vi "IMS Stepper -- V4.vi"() -> ()   [LabVIEW 2018]
doc: "Use this template to build a producer/consumer design pattern with events to produce queue items. Use this design pattern instead of the User Interface Event Handler pattern for user interfaces when you want to execute code asynchronously in response to an event without slowing the user interface responsiveness."
uses:
  publisher action.ctl
  motor internal action.ctl
  slider action.ctl
  slider setter action.ctl
  stepper motor action.ctl
  slider setter interal state.ctl
  stepper motor state.ctl
  internal stepper driver state -- IMS.ctl
  stepper monitor message.ctl
panel:
  in  "Tab Control":enum32{"main", "init&stuff", "ignore"}(tab)
  in  "speed":i32=4003
  in  "stepper state":T1=enum."stopped"
  in  "set angle":dbl(slide)=-10.106382978723403 scale=-56.0..55.0 scale format="%^#6_6g"
  in  "XY Graph":cluster{dbl[], dbl[]}[](graph)=[{[-0.30000000000000004, -0.23550000000000004, -0.17100000000000004, -0.10650000000000004, -0.04200000000000004, 0.022499999999999964, 0.08699999999999997, 0.15149999999999997, 0.21599999999999997, 0.28049999999999997, 0.345, 0.4095, 0.474, 0.5385, 0.603, 0.6675, 0.732, 0.7965, 0.861, 0.9255], [0.0, 0.0, 0.0, 0.0, 0.0, 0.0, 0.0, 0.0, 0.0, 0.0, 0.0, 0.0, 0.0, 0.0, 0.0, 0.0, 0.0, 0.0, 0.0, 0.0]}, {[-0.29607463230851366, -0.23241858636218324, -0.1687625404158528, -0.10510649446952239, -0.04145044852319196, 0.02220559742313849, 0.08586164336946889, 0.14951768931579928, 0.21317373526212974, 0.2768297812084602, 0.34048582715479064, 0.404141873101121, 0.46779791904745144, 0.531453964993782, 0.5951100109401122, 0.6587660568864426, 0.7224221028327731, 0.7860781487791035, 0.849734194725434, 0.9133902406717644], [0.048371604308503874, 0.03797170938217554, 0.02757181445584721, 0.01717191952951888, 0.006772024603190548, -0.0036278703231377857, -0.014027765249466112, -0.024427660175794452, -0.03482755510212278, -0.045227450028451105, -0.055627344954779445, -0.06602723988110777, -0.0764271348074361, -0.08682702973376444, -0.09722692466009278, -0.10762681958642109, -0.11802671451274943, -0.12842660943907777, -0.13882650436540608, -0.14922639929173442]}, {[1.0, 0.9980267284282716, 0.9921147013144779, 0.9822872507286887, 0.9685831611286311, 0.9510565162951535, 0.9297764858882513, 0.9048270524660195, 0.8763066800438636, 0.8443279255020151, 0.8090169943749475, 0.7705132427757891, 0.7289686274214116, 0.6845471059286886, 0.6374239897486896, 0.587785252292473, 0.5358267949789965, 0.48175367410171516, 0.42577929156507266, 0.36812455268467786, 0.30901699437494745, 0.24868988716485474, 0.18738131458572452, 0.12533323356430426, 0.0627905195293133, -1.6081428723391245e-16, -0.0627905195293134, -0.12533323356430437, -0.18738131458572482, -0.24868988716485485, -0.30901699437494756, -0.368124552684678, -0.4257792915650727, -0.48175367410171543, -0.5358267949789969, -0.587785252292473, -0.6374239897486897, -0.6845471059286887, -0.7289686274214117, -0.7705132427757894, -0.8090169943749473, -0.8443279255020151, -0.8763066800438636, -0.9048270524660196, -0.9297764858882515, -0.9510565162951536, -0.9685831611286311, -0.9822872507286887, -0.9921147013144779, -0.9980267284282716, -1.0, -0.9980267284282716, -0.9921147013144779, -0.9822872507286886, -0.9685831611286311, -0.9510565162951535, -0.9297764858882512, -0.9048270524660195, -0.8763066800438635, -0.844327925502015, -0.8090169943749472, -0.770513242775789, -0.7289686274214116, -0.6845471059286886, -0.6374239897486895, -0.5877852522924732, -0.5358267949789963, -0.48175367410171527, -0.42577929156507216, -0.3681245526846778, -0.30901699437494756, -0.24868988716485443, -0.18738131458572463, -0.12533323356430373, -0.06279051952931321, -1.836909530733566e-16, 0.06279051952931372, 0.12533323356430423, 0.18738131458572513, 0.24868988716485493, 0.30901699437494723, 0.36812455268467825, 0.4257792915650726, 0.4817536741017157, 0.5358267949789968, 0.5877852522924737, 0.63742398974869, 0.6845471059286886, 0.7289686274214119, 0.7705132427757894, 0.8090169943749478, 0.8443279255020153, 0.8763066800438636, 0.9048270524660197, 0.9297764858882515, 0.9510565162951538, 0.9685831611286312, 0.9822872507286887, 0.9921147013144779, 0.9980267284282716], [0.0, 0.06279051952931337, 0.12533323356430426, 0.18738131458572463, 0.2486898871648548, 0.3090169943749474, 0.368124552684678, 0.4257792915650727, 0.4817536741017153, 0.5358267949789967, 0.5877852522924731, 0.6374239897486897, 0.6845471059286887, 0.7289686274214116, 0.7705132427757893, 0.8090169943749475, 0.8443279255020151, 0.8763066800438637, 0.9048270524660196, 0.9297764858882515, 0.9510565162951535, 0.9685831611286311, 0.9822872507286887, 0.9921147013144779, 0.9980267284282716, 1.0, 0.9980267284282716, 0.9921147013144778, 0.9822872507286886, 0.9685831611286311, 0.9510565162951535, 0.9297764858882513, 0.9048270524660195, 0.8763066800438635, 0.844327925502015, 0.8090169943749475, 0.7705132427757893, 0.7289686274214114, 0.6845471059286885, 0.6374239897486895, 0.5877852522924732, 0.5358267949789967, 0.4817536741017152, 0.4257792915650725, 0.36812455268467775, 0.3090169943749471, 0.24868988716485482, 0.18738131458572457, 0.1253332335643041, 0.06279051952931314, -3.216285744678249e-16, -0.06279051952931335, -0.12533323356430429, -0.18738131458572477, -0.24868988716485502, -0.30901699437494773, -0.3681245526846783, -0.42577929156507266, -0.4817536741017154, -0.5358267949789968, -0.5877852522924734, -0.63742398974869, -0.6845471059286887, -0.7289686274214116, -0.7705132427757894, -0.8090169943749473, -0.8443279255020153, -0.8763066800438636, -0.9048270524660198, -0.9297764858882515, -0.9510565162951535, -0.9685831611286312, -0.9822872507286887, -0.9921147013144779, -0.9980267284282716, -1.0, -0.9980267284282716, -0.9921147013144779, -0.9822872507286886, -0.9685831611286311, -0.9510565162951536, -0.9297764858882512, -0.9048270524660196, -0.8763066800438634, -0.844327925502015, -0.809016994374947, -0.770513242775789, -0.7289686274214116, -0.6845471059286883, -0.6374239897486896, -0.5877852522924726, -0.5358267949789963, -0.4817536741017153, -0.4257792915650722, -0.36812455268467786, -0.3090169943749468, -0.2486898871648545, -0.18738131458572468, -0.1253332335643038, -0.06279051952931326]}, {[0.1, 0.09980267284282716, 0.0992114701314478, 0.09822872507286888, 0.09685831611286311, 0.09510565162951536, 0.09297764858882514, 0.09048270524660196, 0.08763066800438636, 0.08443279255020152, 0.08090169943749476, 0.07705132427757892, 0.07289686274214116, 0.06845471059286887, 0.06374239897486897, 0.05877852522924731, 0.05358267949789966, 0.04817536741017152, 0.042577929156507266, 0.03681245526846779, 0.030901699437494747, 0.024868988716485477, 0.018738131458572452, 0.012533323356430426, 0.006279051952931331, -1.6081428723391246e-17, -0.0062790519529313405, -0.012533323356430438, -0.018738131458572484, -0.024868988716485487, -0.030901699437494757, -0.0368124552684678, -0.04257792915650727, -0.048175367410171546, -0.05358267949789969, -0.05877852522924731, -0.06374239897486898, -0.06845471059286888, -0.07289686274214117, -0.07705132427757894, -0.08090169943749474, -0.08443279255020152, -0.08763066800438636, -0.09048270524660196, -0.09297764858882515, -0.09510565162951537, -0.09685831611286311, -0.09822872507286888, -0.0992114701314478, -0.09980267284282716, -0.1, -0.09980267284282716, -0.0992114701314478, -0.09822872507286887, -0.09685831611286311, -0.09510565162951536, -0.09297764858882512, -0.09048270524660196, -0.08763066800438635, -0.0844327925502015, -0.08090169943749473, -0.07705132427757891, -0.07289686274214116, -0.06845471059286887, -0.06374239897486896, -0.05877852522924733, -0.05358267949789963, -0.04817536741017153, -0.04257792915650722, -0.036812455268467784, -0.030901699437494757, -0.024868988716485445, -0.018738131458572463, -0.012533323356430374, -0.006279051952931321, -1.836909530733566e-17, 0.006279051952931373, 0.012533323356430424, 0.018738131458572515, 0.024868988716485494, 0.030901699437494726, 0.036812455268467825, 0.042577929156507266, 0.048175367410171574, 0.05358267949789968, 0.05877852522924737, 0.063742398974869, 0.06845471059286887, 0.07289686274214119, 0.07705132427757894, 0.08090169943749478, 0.08443279255020153, 0.08763066800438636, 0.09048270524660197, 0.09297764858882515, 0.09510565162951538, 0.09685831611286312, 0.09822872507286888, 0.0992114701314478, 0.09980267284282716], [0.0, 0.006279051952931338, 0.012533323356430426, 0.018738131458572463, 0.02486898871648548, 0.03090169943749474, 0.0368124552684678, 0.04257792915650727, 0.04817536741017153, 0.05358267949789967, 0.058778525229247314, 0.06374239897486898, 0.06845471059286888, 0.07289686274214116, 0.07705132427757894, 0.08090169943749476, 0.08443279255020152, 0.08763066800438638, 0.09048270524660196, 0.09297764858882515, 0.09510565162951536, 0.09685831611286311, 0.09822872507286888, 0.0992114701314478, 0.09980267284282716, 0.1, 0.09980267284282716, 0.09921147013144778, 0.09822872507286887, 0.09685831611286311, 0.09510565162951536, 0.09297764858882514, 0.09048270524660196, 0.08763066800438635, 0.0844327925502015, 0.08090169943749476, 0.07705132427757894, 0.07289686274214115, 0.06845471059286885, 0.06374239897486896, 0.05877852522924733, 0.05358267949789967, 0.048175367410171525, 0.04257792915650725, 0.03681245526846778, 0.030901699437494712, 0.024868988716485484, 0.01873813145857246, 0.01253332335643041, 0.0062790519529313145, -3.216285744678249e-17, -0.006279051952931335, -0.01253332335643043, -0.018738131458572477, -0.024868988716485504, -0.030901699437494774, -0.03681245526846783, -0.042577929156507266, -0.04817536741017154, -0.05358267949789968, -0.05877852522924734, -0.063742398974869, -0.06845471059286888, -0.07289686274214116, -0.07705132427757894, -0.08090169943749474, -0.08443279255020153, -0.08763066800438636, -0.09048270524660199, -0.09297764858882515, -0.09510565162951536, -0.09685831611286312, -0.09822872507286888, -0.0992114701314478, -0.09980267284282716, -0.1, -0.09980267284282716, -0.0992114701314478, -0.09822872507286887, -0.09685831611286311, -0.09510565162951537, -0.09297764858882512, -0.09048270524660196, -0.08763066800438635, -0.0844327925502015, -0.0809016994374947, -0.07705132427757891, -0.07289686274214116, -0.06845471059286883, -0.06374239897486897, -0.05877852522924726, -0.05358267949789963, -0.04817536741017153, -0.042577929156507224, -0.03681245526846779, -0.03090169943749468, -0.02486898871648545, -0.01873813145857247, -0.012533323356430379, -0.006279051952931327]}, {[0.0, 0.0, 0.0, 0.0, 0.0, 0.0, 0.0, 0.0, 0.0, 0.0, 0.0, 0.0, 0.0, 0.0, 0.0, 0.0, 0.0, 0.0, 0.0, 0.0], [1.1, 1.135, 1.1700000000000002, 1.205, 1.24, 1.2750000000000001, 1.31, 1.345, 1.3800000000000001, 1.415, 1.4500000000000002, 1.485, 1.52, 1.5550000000000002, 1.59, 1.625, 1.6600000000000001, 1.695, 1.73, 1.7650000000000001]}, {[-0.09587131702242406, -0.09674287444990064, -0.09761443187737723, -0.0984859893048538, -0.0993575467323304, -0.10022910415980697, -0.10110066158728355, -0.10197221901476014, -0.10284377644223672, -0.10371533386971331, -0.10458689129718989, -0.10545844872466646, -0.10633000615214305, -0.10720156357961963, -0.10807312100709622, -0.1089446784345728, -0.10981623586204937, -0.11068779328952597, -0.11155935071700254, -0.11243090814447912], [1.0958141679009201, 1.1057761148818375, 1.115738061862755, 1.1257000088436726, 1.13566195582459, 1.1456239028055073, 1.1555858497864249, 1.1655477967673424, 1.1755097437482598, 1.1854716907291771, 1.1954336377100947, 1.2053955846910123, 1.2153575316719296, 1.225319478652847, 1.2352814256337645, 1.245243372614682, 1.2552053195955994, 1.2651672665765168, 1.2751292135574344, 1.285091160538352]}, {[-0.09587131702242406, -0.09674287444990064, -0.09761443187737723, -0.0984859893048538, -0.0993575467323304, -0.10022910415980697, -0.10110066158728355, -0.10197221901476014, -0.10284377644223672, -0.10371533386971331, -0.10458689129718989, -0.10545844872466646, -0.10633000615214305, -0.10720156357961963, -0.10807312100709622, -0.1089446784345728, -0.10981623586204937, -0.11068779328952597, -0.11155935071700254, -0.11243090814447912], [-1.0958141679009201, -1.1057761148818375, -1.115738061862755, -1.1257000088436726, -1.13566195582459, -1.1456239028055073, -1.1555858497864249, -1.1655477967673424, -1.1755097437482598, -1.1854716907291771, -1.1954336377100947, -1.2053955846910123, -1.2153575316719296, -1.225319478652847, -1.2352814256337645, -1.245243372614682, -1.2552053195955994, -1.2651672665765168, -1.2751292135574344, -1.285091160538352]}]
  out "cur angle":dbl(slide)=-9.278801002424245 scale=-95.0..95.0 scale format="%^#6_6g"
  in  "set step !":dbl(slide)=7372.340425531916 min=0.0 max=16000.0 scale=0.0..16500.0 scale format="%^#6_6g"
  out "cur step":dbl(slide)=7444.209386631578 scale=0.0..16500.0
  in  "Go!":bool
  in  "Stop!":bool
  in  "set speed!!":bool
  out "-- exit sync":bool
  in  "Instrument Address":refnum<visa-resource-name>="ASRL2::INSTR"
  in  "Set to zero!":bool
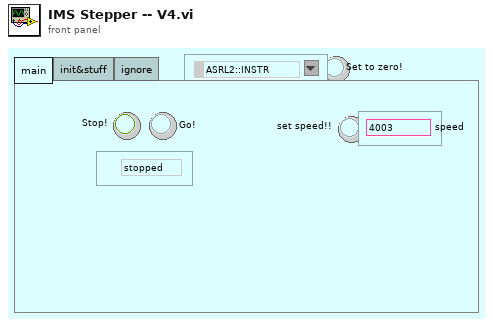
[diagram p1: front panel]
types:
  T1 = typedef "stepper motor state.ctl" = enum16{"moving", "stopped"}
  T2 = typedef "stepper monitor message.ctl" = cluster{"current position":dbl, "stepper motor state OUT":T1}
  T3 = typedef "internal stepper driver state -- IMS.ctl" = cluster{"VISA address":refnum<visa-resource-name>, "stepper motor state":T1, "Motor Address":u32, "speed":i32, "target position":dbl, "current position":dbl}
  T4 = typedef "stepper motor action.ctl" = enum16{"go", "void", "stop", "check", "init", "sync", "set", "set speed", "--check status", "--check value"}
  T5 = typedef "slider setter interal state.ctl" = cluster{"set pos slider":refnum<vi>, "cur angle slider":refnum<vi>, "current pos... slider":refnum<vi>, "XY Graph":refnum<vi>, "set angle":dbl, "pos angle":dbl, "set angle slider":refnum<vi>}
  T6 = typedef "slider setter action.ctl" = enum16{"--update circle", "set step slider moves", "cursor moves", "current pos changed", "init", "void", "--draw current lie", "--draw set line", "--move current step slider", "--move set step slider", "--draw limit lines", "check", "--move set angle slider", "--move current angle slider", "set angle slider moves", "--move cursor", "set set step", "set current step"}
  T7 = typedef "motor internal action.ctl" = enum16{"set slider moves", "update scale", "exit", "current positon changed", "stop", "go", "set speed", "set to zero", "sync"}
  T8 = typedef "publisher action.ctl" = enum16{"set", "get"}
  T9 = typedef "slider action.ctl" = enum16{"check", "copy range", "set from value", "set from ratio", "set from slider", "read using other slider"}
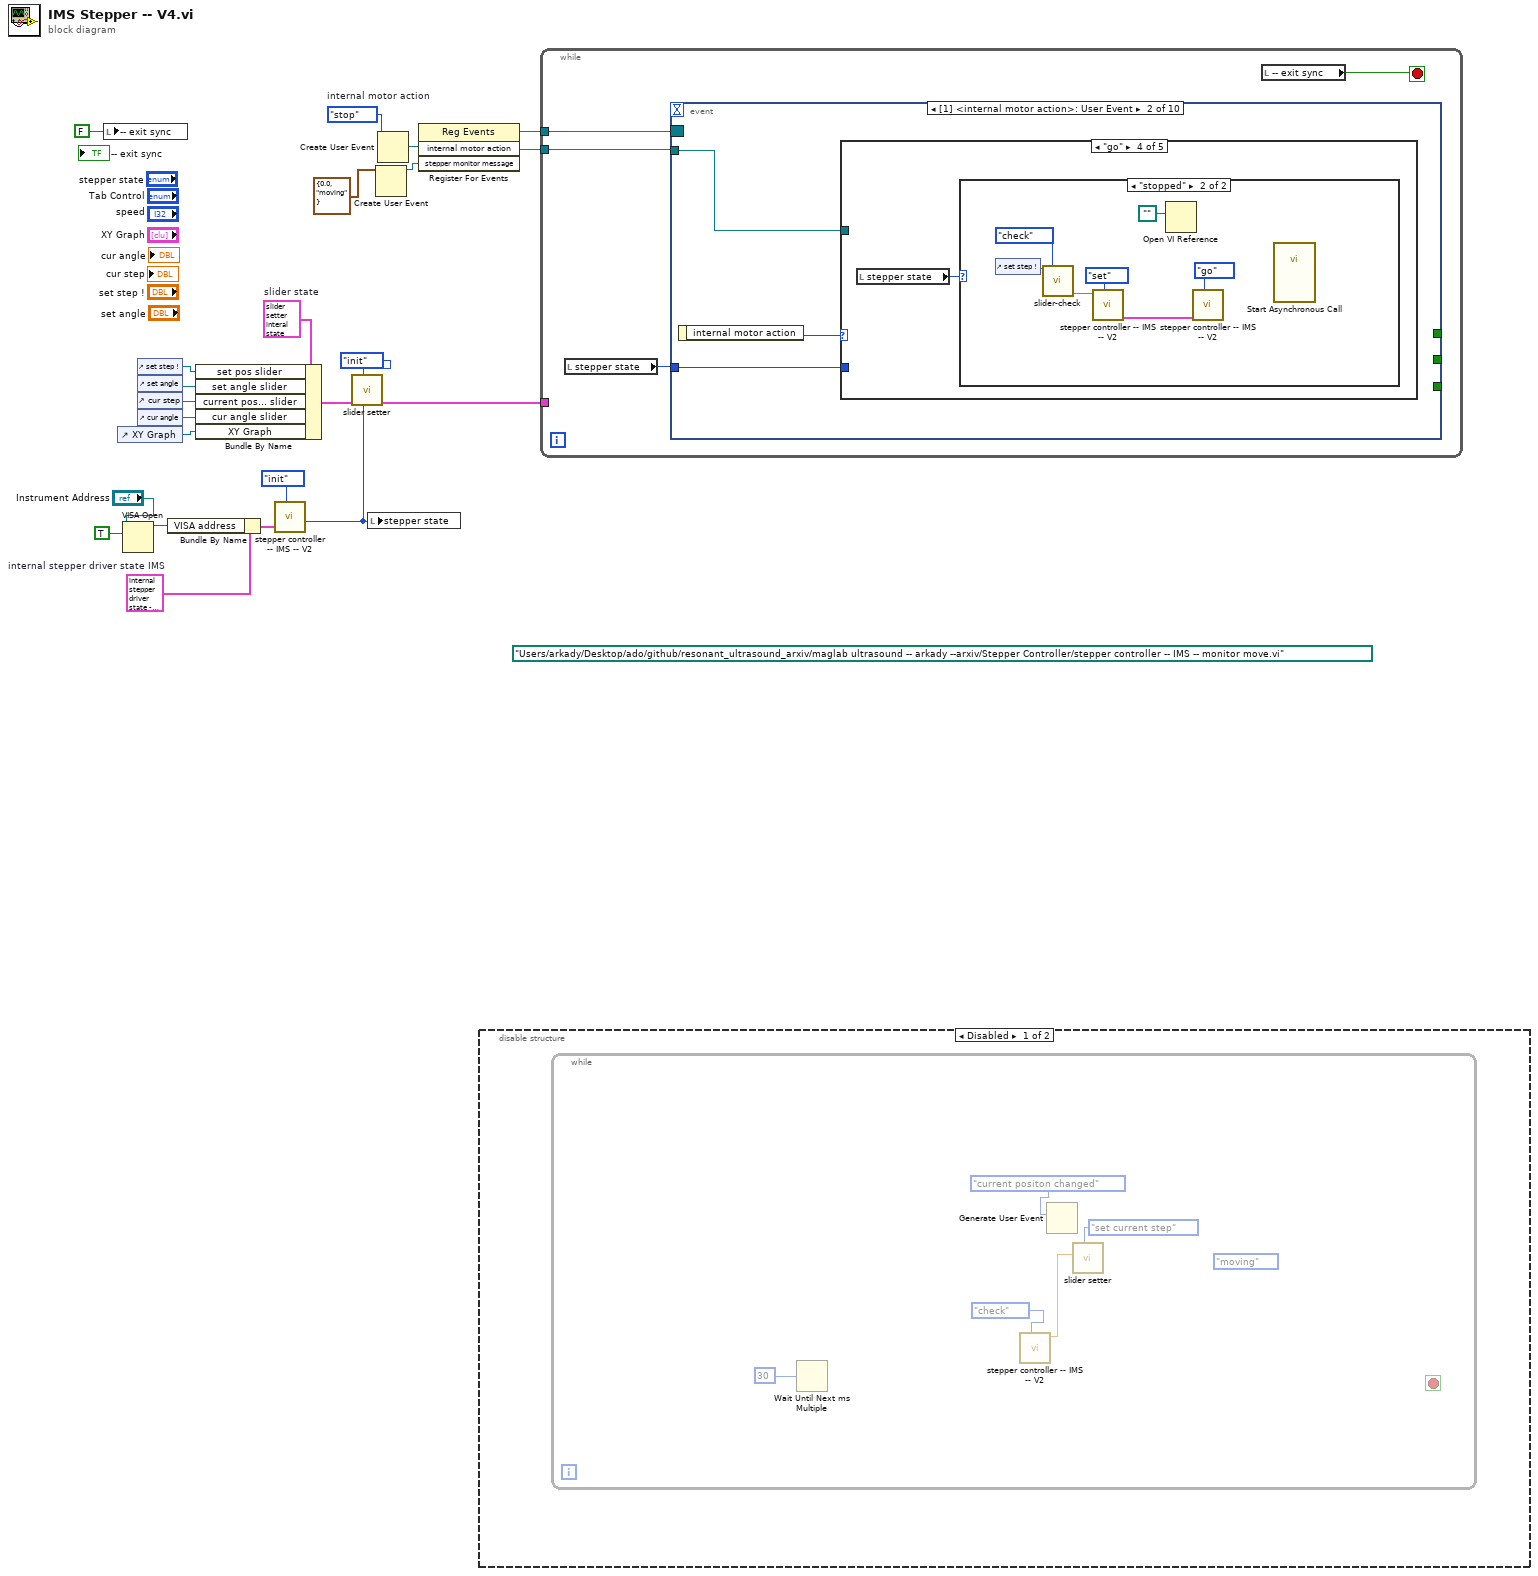
[diagram p0: block diagram]
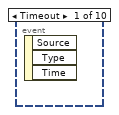
[diagram p3: hidden frame]
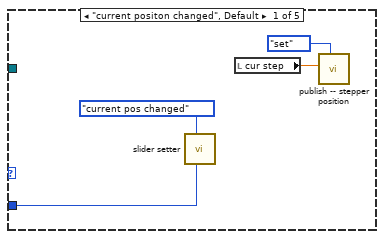
[diagram p4: hidden frame]
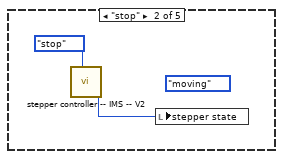
[diagram p5: hidden frame]
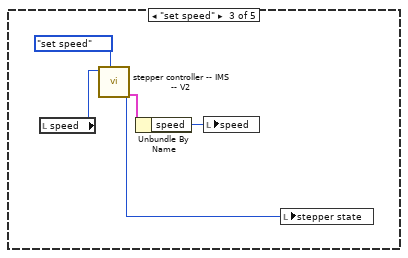
[diagram p6: hidden frame]
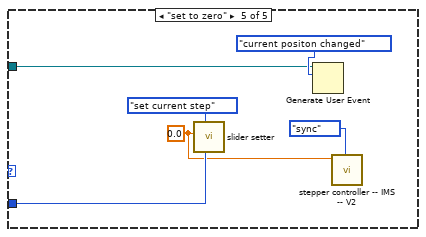
[diagram p8: hidden frame]
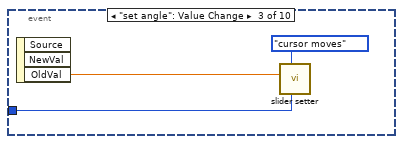
[diagram p9: hidden frame]
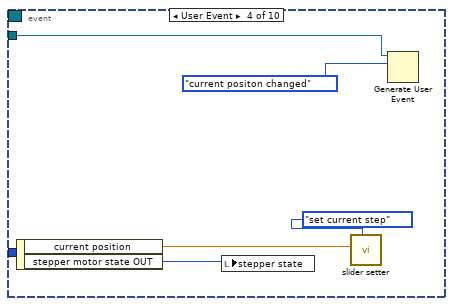
[diagram p10: hidden frame]
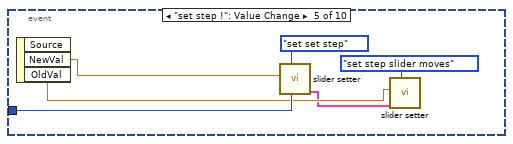
[diagram p11: hidden frame]
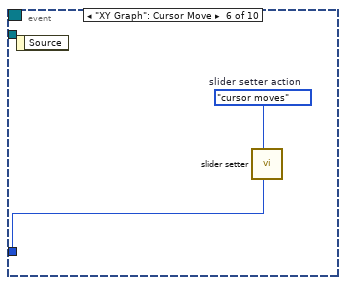
[diagram p12: hidden frame]
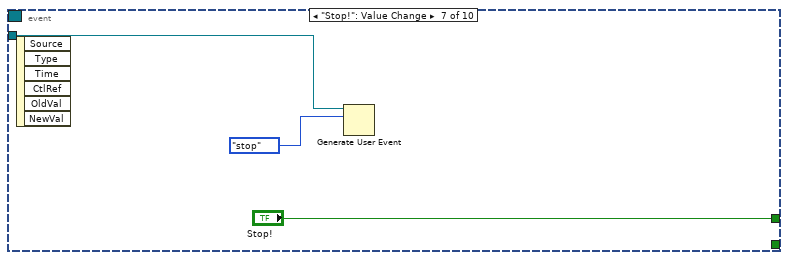
[diagram p13: hidden frame]
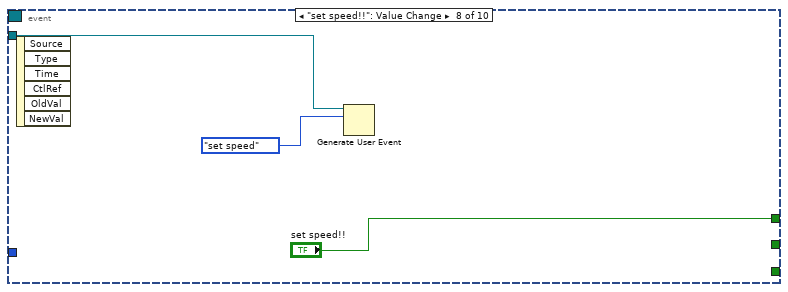
[diagram p14: hidden frame]
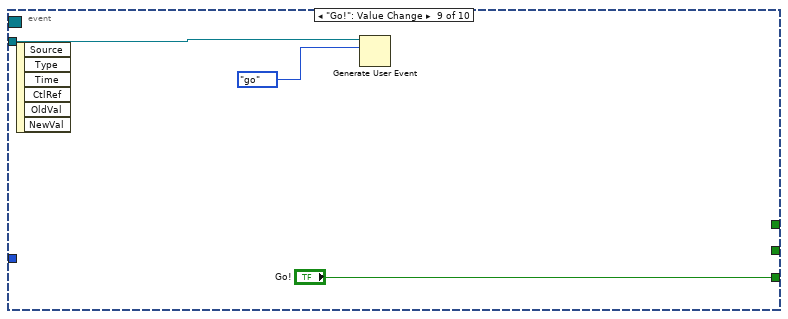
[diagram p15: hidden frame]
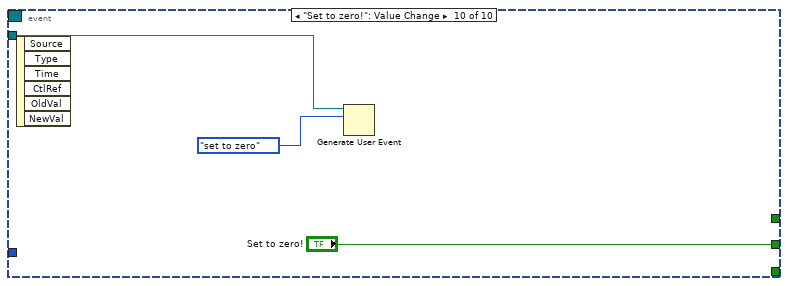
[diagram p16: hidden frame]
diagram:
  (unwired) path "/Users/arkady/Desktop/ado/github/resonant_ultrasound_arxiv/maglab ultrasound -- arkady --arxiv/Stepper Controller/stepper controller -- IMS -- monitor move.vi" ("vi path")
  w4 = T3 {"VISA address"="GPIB0::25::INSTR", "stepper motor state"=enum."stopped", "Motor Address"=0, "speed"=0, "target position"=0.0, "current position"=0.0}  # internal stepper driver state IMS
  w17 = T5 {"set pos slider"=refnum, "cur angle slider"=refnum, "current pos... slider"=refnum, "XY Graph"=refnum, "set angle"=0.0, "pos angle"=0.0, "set angle slider"=refnum}  # slider state
  w19 = motor_internal_action."stop"  # internal motor action
  n1 = local write "-- exit sync"(FALSE ("-- exit  signal")) -> ()
  n2 = control-ref of="XY Graph"() -> (w16:refnum<vi>)
  n3 = VISA Open(duplicate session (F)=TRUE, VISA resource name="Instrument Address") -> (VISA resource name=w8:refnum<visa-resource-name>)  [unwired: 3 in, 1 out]
  n4 = control-ref of="set step !"() -> (w12:refnum<vi>)
  n5 = control-ref of="set angle"() -> (w13:refnum<vi>)
  n6 = control-ref of="cur step"() -> (w14:refnum<vi>)
  n7 = control-ref of="cur angle"() -> (w15:refnum<vi>)
  n8 = Bundle By Name(cluster=w4, "VISA address"=w8) -> (w5:T3)
  n9 = Bundle By Name(cluster=w17, "set pos slider"=w12, "set angle slider"=w13, "current pos... slider"=w14, "cur angle slider"=w15, "XY Graph"=w16) -> (w11:T5)
  n10 = call "stepper controller -- IMS -- V2.vi"("stepper driver action"=stepper_motor_action."init", "internal stepper driver state IMS"=w5) -> ("stepper motor state OUT"=w3:T1)  [unwired: 7 in, 2 out]
  n11 = call "slider setter.vi"("stepper motor state"=w3, "slider setter action"=slider_setter_action."init", "state in"=w11) -> ("state OUT"=w10:T5)  [unwired: 8 in]
  n12 = local write "stepper state"(w3) -> ()
  n13 = Create User Event(user event datatype=T2 {"current position"=0.0, "stepper motor state OUT"=enum."moving"} ("stepper monitor message")) -> (user event=w2:refnum<user-event>)  [unwired: 1 in, 1 out]
  n14 = Create User Event(user event datatype=w19) -> (user event=w7:refnum<user-event>)  [unwired: 1 in, 1 out]
  n15 = register-events(w7, w2) -> (reference out=w20:refnum<event-registration>)  [unwired: 2 in, 1 out]
  n16 = disable-structure shown="Disabled" {
    frame Disabled {
      n17 = while {
        stop <- _ stop-if-true
        (unwired) stepper_motor_state."moving" ("stepper motor state OUT")
        n18 = Wait Until Next ms Multiple(millisecond multiple=u32 30) -> ()  [unwired: 1 out]
        n19 = call "stepper controller -- IMS -- V2.vi"("stepper driver action"=stepper_motor_action."check") -> ("current position"=w27:dbl)  [unwired: 8 in, 2 out]
        n20 = Generate User Event(event data cluster=motor_internal_action."current positon changed" ("event data")) -> ()  [unwired: 3 in, 2 out]
        n21 = call "slider setter.vi"("slider setter action"=slider_setter_action."set current step", "value"=w27) -> ()  [unwired: 9 in, 1 out]
      }
    }
    frame Enabled {
    }
  }
  n22 = while {
    tunnel: w20 -> [w31]
    tunnel: w7 -> [w30]
    tunnel: w10 -> [_]
    stop <- w28 stop-if-true
    n23 = local read "stepper state"() -> (w29:T1)
    n24 = event shown="[1] <internal motor action>: User Event" {
      selector: w31 -> [_ _ _ _ _ _ _ _ _ _]
      dyn-events: _ -> [_ _ _ _ _ _ _ _ _ _]
      timeout: _ -> [_ _ _ _ _ _ _ _ _ _]
      tunnel: w30 -> [_ w32 _ w64 _ _ w77 w81 w84 w87]
      tunnel: w29 -> [_ w33 w60 _ w72 w74 _ _ _ _]
      tunnel: [_ _ _ _ _ _ "Stop!" "set speed!!" _ _] -> _
      tunnel: [_ _ _ _ _ _ _ _ "Go!" _] -> _
      tunnel: [_ _ _ _ _ _ _ _ _ "Set to zero!"] -> _
      event Timeout {
        n25 = event-data() -> ()  [unwired: 1 in, 3 out]
      }
      event User Event {
        n26 = event-data() -> ("internal motor action"=w34:T7)  [unwired: 1 in]
        n27 = case shown="\"go\"" w34 {
          tunnel: w33 -> [w35 _ _ _ w58]
          tunnel: w32 -> [_ _ _ _ w56]
          frame "current positon changed", Default {
            n28 = call "slider setter.vi"("stepper motor state"=w35, "slider setter action"=slider_setter_action."current pos changed") -> ()  [unwired: 9 in, 1 out]
            n29 = local read "cur step"() -> (w37:dbl)
            n30 = call "publish -- stepper position.vi"("publisher action"=publisher_action."set", "stepper pos IN"=w37) -> ()  [unwired: 9 in, 1 out]
          }
          frame "stop" {
            (unwired) stepper_motor_state."moving" ("stepper motor state OUT")
            n31 = call "stepper controller -- IMS -- V2.vi"("stepper driver action"=stepper_motor_action."stop") -> ("stepper motor state OUT"=w39:T1)  [unwired: 8 in, 2 out]
            n32 = local write "stepper state"(w39) -> ()
          }
          frame "set speed" {
            n33 = local read "speed"() -> (w43:i32)
            n34 = call "stepper controller -- IMS -- V2.vi"("stepper driver action"=stepper_motor_action."set speed", "number"=w43) -> ("internal stepper driver state IMS -- OUT"=w42:T3, "stepper motor state OUT"=w44:T1)  [unwired: 7 in, 1 out]
            n35 = Unbundle By Name(w42) -> ("speed"=w41:i32)
            n36 = local write "speed"(w41) -> ()
            n37 = local write "stepper state"(w44) -> ()
          }
          frame "go" {
            n38 = local read "stepper state"() -> (w46:T1)
            n39 = case shown="\"stopped\"" w46 {
              frame "moving", Default {
              }
              frame "stopped" {
                n40 = control-ref of="set step !"() -> (w52:refnum<vi>)
                n41 = call "slider-check.vi"("slider"=w52, "slider action"=slider_action."check") -> ("value OUT"=w50:dbl)  [unwired: 9 in, 4 out]
                n42 = call "stepper controller -- IMS -- V2.vi"("stepper driver action"=stepper_motor_action."set", "number"=w50) -> ("internal stepper driver state IMS -- OUT"=w48:T3)  [unwired: 7 in, 2 out]
                n43 = Open VI Reference(vi path=path "") -> ()  [unwired: 5 in, 2 out]
                n44 = call "stepper controller -- IMS -- V2.vi"("stepper driver action"=stepper_motor_action."go", "internal stepper driver state IMS"=w48) -> ()  [unwired: 7 in, 3 out]
                n45 = call-by-ref "Start Asynchronous Call"() -> ()  [unwired: 2 in, 2 out]
              }
            }
          }
          frame "set to zero" {
            w54 = 0.0 ("value")
            n46 = call "slider setter.vi"("stepper motor state"=w58, "slider setter action"=slider_setter_action."set current step", "value"=w54) -> ()  [unwired: 8 in, 1 out]
            n47 = Generate User Event(user event=w56, event data cluster=motor_internal_action."current positon changed" ("event data")) -> ()  [unwired: 2 in, 2 out]
            n48 = call "stepper controller -- IMS -- V2.vi"("stepper driver action"=stepper_motor_action."sync", "number"=w54) -> ()  [unwired: 7 in, 3 out]
          }
        }
      }
      event "set angle": Value Change {
        n49 = event-data() -> ("OldVal"=w62:dbl)  [unwired: 1 in, 2 out]
        n50 = call "slider setter.vi"("stepper motor state"=w60, "slider setter action"=slider_setter_action."cursor moves", "value"=w62) -> ()  [unwired: 8 in, 1 out]
      }
      event User Event {
        n51 = event-data() -> ("current position"=w66:dbl, "stepper motor state OUT"=w65:T1)  [unwired: 1 in]
        n52 = local write "stepper state"(w65) -> ()
        n53 = call "slider setter.vi"("slider setter action"=slider_setter_action."set current step", "value"=w66) -> ()  [unwired: 9 in, 1 out]
        n54 = Generate User Event(user event=w64, event data cluster=motor_internal_action."current positon changed" ("event data")) -> ()  [unwired: 2 in, 2 out]
      }
      event "set step !": Value Change {
        n55 = event-data() -> ("NewVal"=w70:dbl, "OldVal"=w69:dbl)  [unwired: 1 in, 1 out]
        n56 = call "slider setter.vi"("stepper motor state"=w72, "slider setter action"=slider_setter_action."set set step", "value"=w70) -> ("state OUT"=w68:T5)  [unwired: 8 in]
        n57 = call "slider setter.vi"("slider setter action"=slider_setter_action."set step slider moves", "state in"=w68, "value"=w69) -> ()  [unwired: 8 in, 1 out]
      }
      event "XY Graph": Cursor Move {
        w75 = slider_setter_action."cursor moves"  # slider setter action
        n58 = event-data() -> ()  [unwired: 1 in, 1 out]
        n59 = call "slider setter.vi"("stepper motor state"=w74, "slider setter action"=w75) -> ()  [unwired: 9 in, 1 out]
      }
      event "Stop!": Value Change {
        n60 = event-data() -> ()  [unwired: 1 in, 6 out]
        n61 = Generate User Event(user event=w77, event data cluster=motor_internal_action."stop" ("event data")) -> ()  [unwired: 2 in, 2 out]
      }
      event "set speed!!": Value Change {
        n62 = event-data() -> ()  [unwired: 1 in, 6 out]
        n63 = Generate User Event(user event=w81, event data cluster=motor_internal_action."set speed" ("event data")) -> ()  [unwired: 2 in, 2 out]
      }
      event "Go!": Value Change {
        n64 = event-data() -> ()  [unwired: 1 in, 6 out]
        n65 = Generate User Event(user event=w84, event data cluster=motor_internal_action."go" ("event data")) -> ()  [unwired: 2 in, 2 out]
      }
      event "Set to zero!": Value Change {
        n66 = event-data() -> ()  [unwired: 1 in, 6 out]
        n67 = Generate User Event(user event=w87, event data cluster=motor_internal_action."set to zero" ("event data")) -> ()  [unwired: 2 in, 2 out]
      }
    }
    n68 = local read "-- exit sync"() -> (w28:bool)
  }
